vi "Write Limit Volt.vi"(8 "error in":errorcluster, 10 "OverVoltage_Protect":dbl, 11 "79XRP in":refnum<class "79XRP.lvclass">) -> (0 "error out":errorcluster, 3 "79XRP out":refnum<class "79XRP.lvclass">)   [LabVIEW 2019, in "79XRP.lvlib" / "79XRP.lvclass"]
uses:
  Library/79XRP.lvclass
  builds/Instruments/PowerSupply.lvlibp/Library/PowerSupply.lvclass
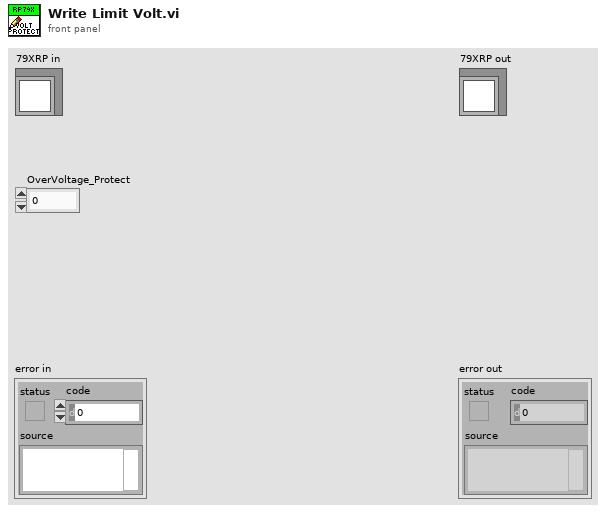
[diagram p1: front panel]
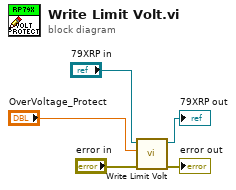
[diagram p0: block diagram]
diagram:
  n1 = call-parent "Write Limit Volt.vi"("error in"="error in", "OverVoltage_Protect"="OverVoltage_Protect", "PowerSupply in"="79XRP in") -> ("error out"=→"error out":errorcluster, "PowerSupply out"=→"79XRP out":refnum<class "79XRP.lvclass">)  [unwired: 7 in]
